vi "get_total_number_of_lines.vi"(8 "error in (no error)":errorcluster, 11 "TrajectoryDL090201FrameScan in":refnum<class "TrajectoryDL090201FrameScan.lvclass">) -> (0 "error out":errorcluster, 2 "total number of y lines":i32, 3 "TrajectoryDL090201FrameScan out":refnum<class "TrajectoryDL090201FrameScan.lvclass">)   [LabVIEW 2010, in "TrajectoryDL090201FrameScan.lvclass"]
uses:
  TrajectoryDL090201FrameScan.lvclass
  TrajectoryDL090201FrameScan.lvclass/TrajectoryDL090201FrameScan.ctl
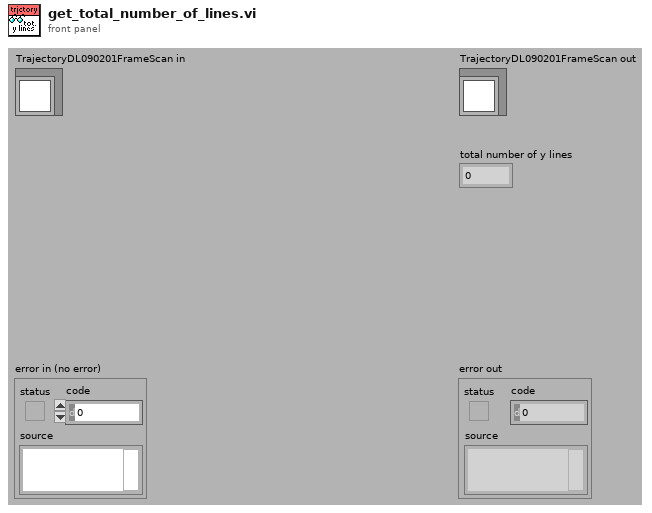
[diagram p1: front panel]
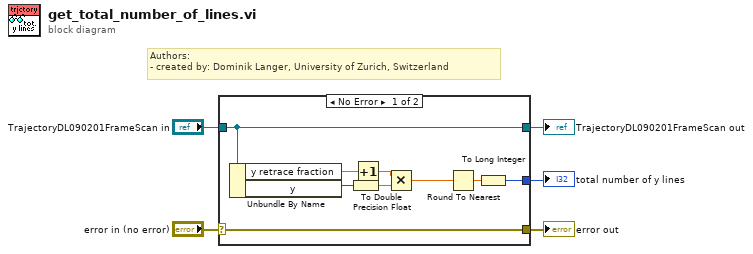
[diagram p0: block diagram]
diagram:
  # "Authors: \n- created by: Dominik Langer, University of Zurich, Switzerland"
  n1 = case shown="No Error" "error in (no error)" {
    selector: "error in (no error)" -> [w14 w16]
    tunnel: [w14 w16] -> w4
    tunnel: [w13 w15] -> w2
    tunnel: "TrajectoryDL090201FrameScan in" -> [w13 w15]
    tunnel: [w6 _] -> w1
    frame No Error {
      n2 = Unbundle By Name(w13) -> ("y retrace fraction"=w10:dbl, "y"=w12:i32)
      n3 = To Double Precision Float(number=w12) -> (double precision float=w11:dbl)
      n4 = Increment(x=w10) -> (x+1=w9:dbl)
      n5 = Multiply(x=w9, y=w11) -> (x*y=w8:dbl)
      n6 = Round To Nearest(number=w8) -> (nearest integer value=w7:dbl)
      n7 = To Long Integer(number=w7) -> (32bit integer=w6:i32)
    }
    frame Error {
    }
  }
  "error out" <- w4
  "TrajectoryDL090201FrameScan out" <- w2
  "total number of y lines" <- w1
